vi "FTW-Collection-Merge.vi"(0 "Collection":refnum<class "FTW-Collection.lvclass">, 5 "Collection to Merge":refnum<class "FTW-Collection.lvclass">, 11 "error in":errorcluster) -> (4 "Collection out":refnum<class "FTW-Collection.lvclass">, 15 "error out":errorcluster)   [LabVIEW 2012, in "FTW-Collection.lvclass"]
uses:
  FTW-Collection.lvclass
panel:
  # "Inputs"
  # "Outputs"
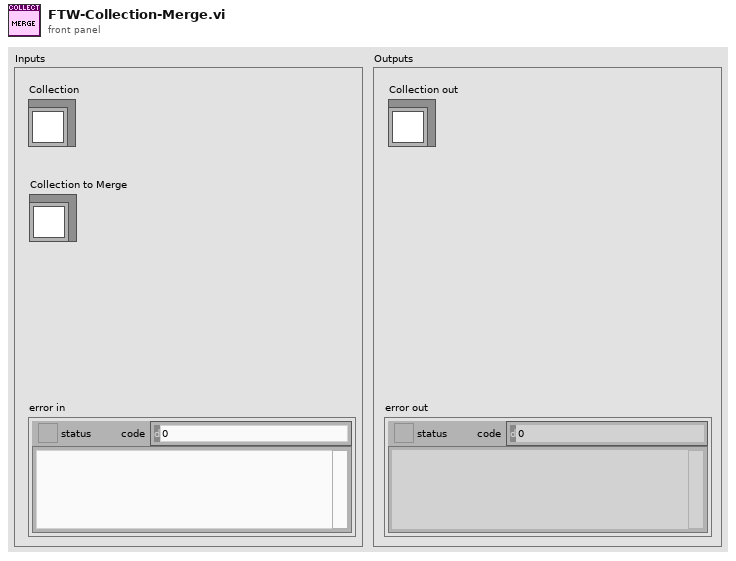
[diagram p1: front panel]
types:
  T1 = typedef "FTW-Collection-KeyVariantPair.ctl" = cluster{"Key":string, "Value":variant}
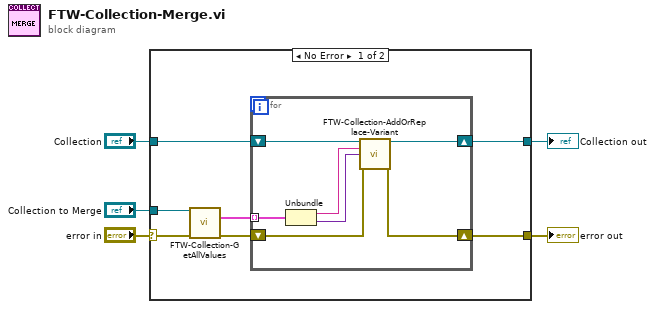
[diagram p0: block diagram]
diagram:
  n1 = case shown="No Error" "error in" {
    selector: "error in" -> [w9 w21]
    tunnel: [w10 w21] -> w5
    tunnel: "Collection" -> [w12 w20]
    tunnel: [w11 w20] -> w2
    tunnel: "Collection to Merge" -> [w6 _]
    frame No Error {
      n2 = call "FTW-Collection-GetAllValues.vi"("Collection"=w6, "error in"=w9) -> ("Key-Variant Pairs"=w7:T1[], "error out"=w8:errorcluster)  [unwired: 11 in, 1 out]
      n3 = for {
        shift-right: [w18] -> w11
        shift-left: w12 -> [w19]
        shift-right: [w17] -> w10
        shift-left: w8 -> [w16]
        tunnel: w7 -> [w15] mode=indexing
        n4 = Unbundle(w15) -> ("Key"=w14:string, "Value"=w13:variant)
        n5 = call "FTW-Collection-AddOrReplace-Variant.vi"("Collection"=w19, "Key"=w14, "Value"=w13, "error in"=w16) -> ("Collection out"=w18:refnum<class "FTW-Collection.lvclass">, "error out"=w17:errorcluster)  [unwired: 9 in, 1 out]
      }
    }
    frame Error {
    }
  }
  "error out" <- w5
  "Collection out" <- w2
